vi "set_intensity_array_old.vi"() -> ()   [LabVIEW 2010, in "FPGAWrapperAK101022Resonance.lvclass"]
uses:
  FPGAWrapperAK101022Resonance.lvclass
  class_data.vi
  z-intensity array.ctl
panel:
  out "FPGA_AK101022Resonance out":refnum<class "FPGAWrapperAK101022Resonance.lvclass">
  in  "FPGA_AK101022Resonance in":refnum<class "FPGAWrapperAK101022Resonance.lvclass">
  out "error out":errorcluster
  in  "error in (no error)":errorcluster
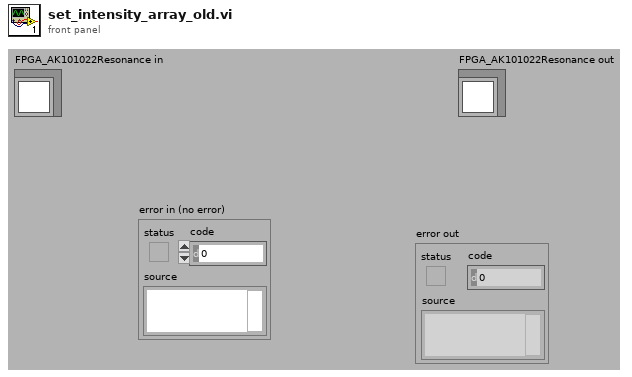
[diagram p1: front panel]
types:
  T1 = typedef "z-intensity array.ctl" = u32[]
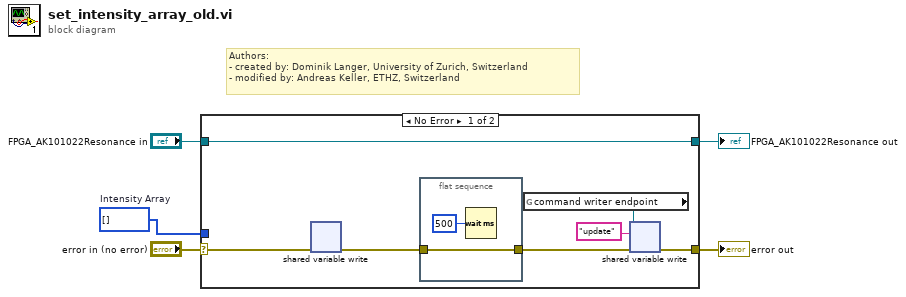
[diagram p0: block diagram]
diagram:
  w1 = T1 []  # Intensity Array
  # "Authors: \n- created by: Dominik Langer, University of Zurich, Switzerland\n- modified by: Andreas Keller, ETHZ, Switzerland"
  n1 = case shown="No Error" "error in (no error)" {
    selector: "error in (no error)" -> [w7 w17]
    tunnel: [w12 w17] -> w3
    tunnel: [w13 w16] -> w2
    tunnel: "FPGA_AK101022Resonance in" -> [w13 w16]
    tunnel: w1 -> [w8 _]
    frame No Error {
      n2 = shared-variable-write(w7) -> (w6:errorcluster)  [unwired: 3 in, 2 out]
      n3 = flat-sequence {
        tunnel: w6 -> [w14]
        tunnel: [w14] -> w9
        frame #0 {
          n4 = Wait (ms)(milliseconds to wait=u32 500) -> ()  [unwired: 1 out]
        }
      }
      n5 = global read "class_data.vi" "command writer endpoint"() -> (w11:refnum<k21>)
      n6 = shared-variable-write(w11, w9, "update" ("data in")) -> (w12:errorcluster)  [unwired: 1 in, 2 out]
    }
    frame Error {
    }
  }
  "error out" <- w3
  "FPGA_AK101022Resonance out" <- w2
